vi "fgt get controllers info.vi"(8 "error in (no error)":errorcluster) -> (0 "error out":errorcluster, 3 "Controllers channels info":T1[](array[typedef]))   [LabVIEW 2020, in "fgt_SDK.lvlib"]
doc: "Retrieve information about session controllers. Controllers are MFCS, Flowboard, Link, IPS in an array."
uses:
  fgt_SDK.lvlib
  TypeDefs/fgt_CONTROLLER_INFO.ctl
  TypeDefs/fgt_INSTRUMENT_TYPE.ctl
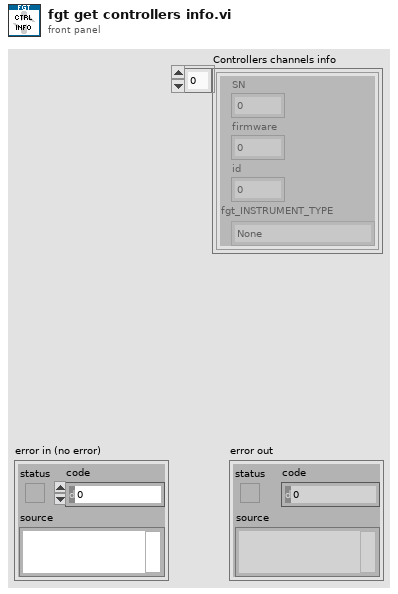
[diagram p1: front panel]
types:
  T1 = typedef "fgt_SDK.lvlib/fgt_CONTROLLER_INFO.ctl" = cluster{"SN":u16, "firmware":u16, "id":u32, "fgt_INSTRUMENT_TYPE":T2}
  T2 = typedef "fgt_SDK.lvlib/fgt_INSTRUMENT_TYPE.ctl" = enum32{"None", "MFCS", "MFCS_EZ", "FRP", "LineUP", "IPS"}
  T3 = typedef "fgt_SDK.lvlib/fgt_STATUS_INFO.ctl" = cluster{"InstrType":T2, "instrSN":u16, "errorCode":u8, "infoCode":u8, "detail":string}
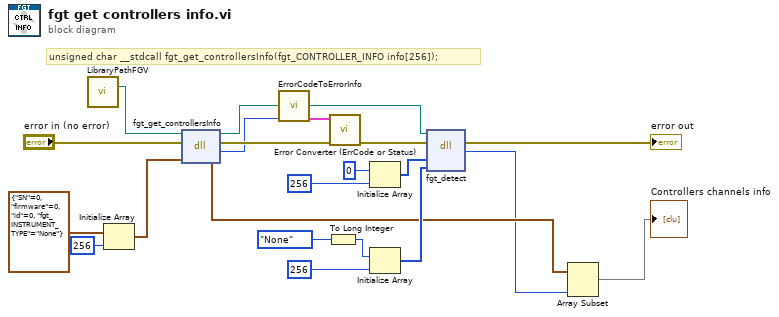
[diagram p0: block diagram]
diagram:
  # "unsigned char __stdcall fgt_get_controllersInfo(fgt_CONTROLLER_INFO info[256]);"
  n1 = call "LibraryPathFGV.vi"() -> ("Path Out"=w2:path)  [unwired: 14 in, 1 out]
  n2 = Initialize Array(T1 {"SN"=0, "firmware"=0, "id"=0, "fgt_INSTRUMENT_TYPE"=enum."None"} ("fgt_CONTROLLER_INFO"), 256 ("dimension size")) -> (w15:T1[])
  n3 = dll-call lib="C:/Workspace/fgt-SDK/LabVIEW/dlls/fgt_SDK_*.*" fn="fgt_get_controllersInfo"(path in=w2, error in="error in (no error)", "info"=w15) -> (path out=w1:path, error out=w20:errorcluster, "return type"=w19:u8, "info"=w5:T1[])  [unwired: 1 in]
  n4 = call "ErrorCodeToErrorInfo.vi"("return type"=w19) -> ("StatusInfo"=w18:T3)  [unwired: 10 in]
  n5 = To Long Integer(number=fgt_INSTRUMENT_TYPE."None" ("fgt_INSTRUMENT_TYPE")) -> (32bit integer=w9:i32)
  n6 = call "Error Converter (ErrCode or Status).vi"("error in (no error)"=w20, "StatusInfo"=w18) -> ("error out"=w7:errorcluster)  [unwired: 9 in]
  n7 = Initialize Array(u16 0 ("element"), 256 ("dimension size")) -> (w8:u16[])
  n8 = Initialize Array(w9, 256 ("dimension size")) -> (w11:i32[])
  n9 = dll-call lib="C:/Workspace/fgt-SDK/LabVIEW/dlls/fgt_SDK_*.*" fn="fgt_detect"(path in=w1, error in=w7, "SN"=w8, "type"=w11) -> (error out=→"error out":errorcluster, "return type"=w3:u8)  [unwired: 3 in, 1 out]
  n10 = Array Subset(array=w5, length=w3) -> (→"Controllers channels info":T1[])  [unwired: 1 in]
